vi "Turn Off Linearization Bins.vi"(10 "Number of Samples":i32, 11 "Number of Pixels":i32) -> (2 "Pre Binned Values":u32[](array[numeric]), 3 "Equal Edges Array":bool[](array[boolean]))   [LabVIEW 2014]
panel:
  out "sum 2":i16
  out "sum":i16
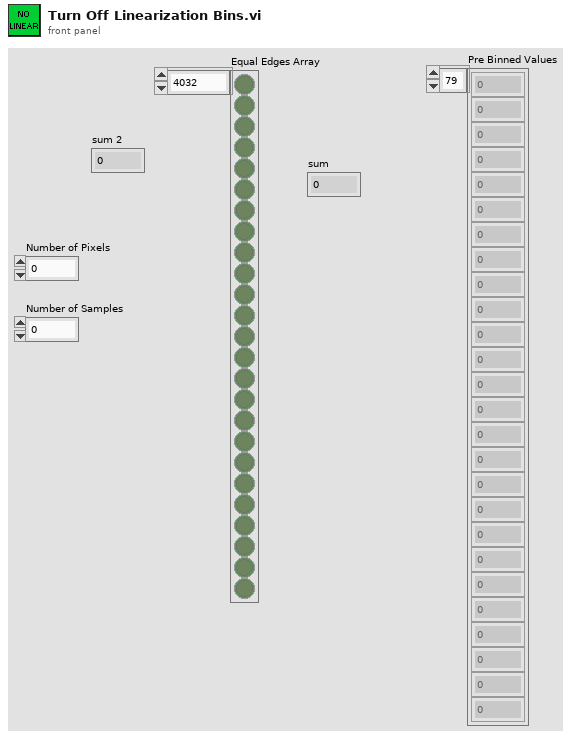
[diagram p1: front panel]
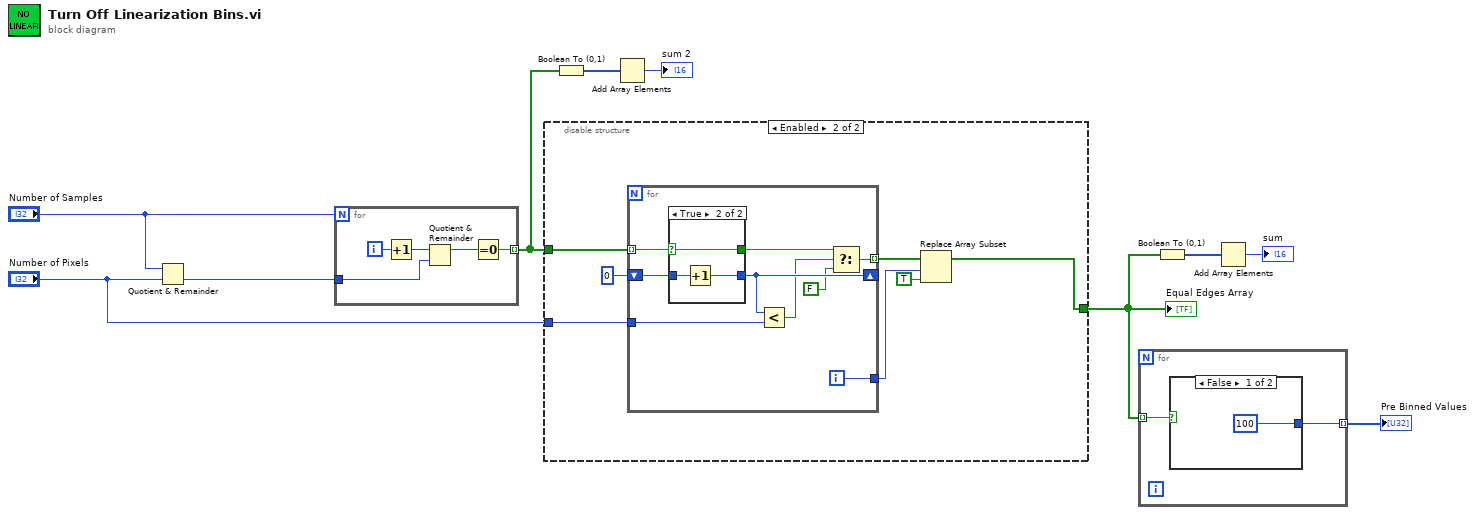
[diagram p0: block diagram]
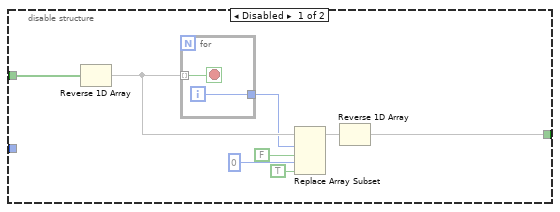
[diagram p2: hidden frame]
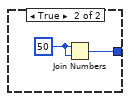
[diagram p4: hidden frame]
diagram:
  n1 = Quotient & Remainder(x="Number of Samples", y="Number of Pixels") -> (floor(x/y)=w2:i32)  [unwired: 1 out]
  n2 = for {
    N: "Number of Samples" -> [_]
    tunnel: w2 -> [w14]
    tunnel: [w11] -> w3 mode=indexing
    i -> [w15]
    n3 = Increment(x=w15) -> (x+1=w12:i32)
    n4 = Quotient & Remainder(x=w12, y=w14) -> (x-y*floor(x/y)=w13:i32)  [unwired: 1 out]
    n5 = Equal To 0?(x=w13) -> (x = 0?=w11:bool)
  }
  n6 = disable-structure shown="Enabled" {
    disable-tunnel: w3 -> [w23 w30]
    disable-tunnel: [w16 w26] -> w8
    disable-tunnel: "Number of Pixels" -> [_ w31]
    frame Disabled {
      n7 = Reverse 1D Array(array=w23) -> (reversed array=w22:bool[])
      n8 = for {
        tunnel: w22 -> [w25] mode=indexing
        tunnel: [w24] -> w21
        i -> [w24]
        stop <- w25 stop-if-true
      }
      n9 = Replace Array Subset(array=w22, new element #1=FALSE ("new element/subarray"), index #1=w21, new element #2=TRUE ("new element/subarray"), index #2=0 ("index")) -> (w17:bool[])
      n10 = Reverse 1D Array(array=w17) -> (reversed array=w16:bool[])
    }
    frame Enabled {
      n11 = for {
        tunnel: w30 -> [w41] mode=indexing
        shift-right: [w39] -> _
        shift-left: 0 -> [w40]
        tunnel: w31 -> [w38]
        tunnel: [w36] -> w29 mode=indexing
        tunnel: [w33] -> w28
        i -> [w33]
        n12 = case shown="True" w41 {
          selector: w41 -> [w43 w44]
          tunnel: w40 -> [w42 w46]
          tunnel: [w42 w45] -> w39
          tunnel: [w43 w44] -> w37
          frame False {
          }
          frame True {
            n13 = Increment(x=w46) -> (x+1=w45:i32)
          }
        }
        n14 = Less?(x=w39, y=w38) -> (x < y?=w35:bool)
        n15 = Select(t=w37, s=w35, f=FALSE) -> (s? t:f=w36:bool)
      }
      n16 = Replace Array Subset(array=w29, new element=TRUE ("new element/subarray"), index=w28) -> (w26:bool[])
    }
  }
  "Equal Edges Array" <- w8
  n17 = Boolean To (0,1)(Boolean=w3) -> (0, 1=w4:i16[])
  n18 = Add Array Elements(numeric array=w4) -> (sum=→"sum 2":i16)
  n19 = for {
    tunnel: w8 -> [w48] mode=indexing
    tunnel: [w47] -> w9 mode=indexing
    n20 = case shown="False" w48 {
      tunnel: [u32 100 w50] -> w47
      frame False {
      }
      frame True {
        w51 = u16 50
        n21 = Join Numbers(hi=w51, lo=w51) -> ((hi.lo)=w50:u32)
      }
    }
  }
  "Pre Binned Values" <- w9
  n22 = Boolean To (0,1)(Boolean=w8) -> (0, 1=w7:i16[])
  n23 = Add Array Elements(numeric array=w7) -> (sum=→"sum":i16)
